vi "Send Initial Position Command.vi"(1 "MCL Command In":refnum<queue>, 2 "Ramp Times":cluster{"Initial":T1, "Iterative":T1}, 3 "error in":errorcluster) -> (5 "MCL Command Out":refnum<queue>, 6 "error out":errorcluster)   [LabVIEW 2009]
uses:
  Mixed Mode Command.ctl
  Mixed Mode Command Action.ctl
  Ramp Time Tuple.ctl
  Target Data.ctl
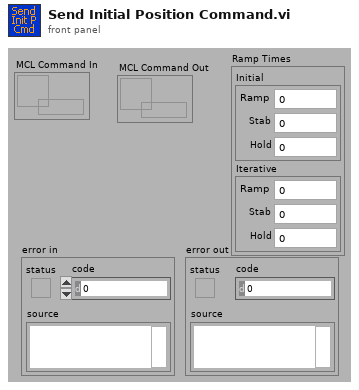
[diagram p1: front panel]
types:
  T1 = typedef "Ramp Time Tuple.ctl" = cluster{"Ramp":dbl, "Stab":dbl, "Hold":dbl}
  T2 = typedef "Mixed Mode Command Action.ctl" = enum16{"Start Command", "Stop", "Exit", "No Op", "Start Acquisition", "Measure Initial Position"}
  T3 = typedef "Mixed Mode Command.ctl" = cluster{"Command":T2, "Ramp Times":cluster{"Initial":T1, "Iterative":T1}, "LBCB1":T4, "LBCB2":T4}
  T4 = typedef "Target Data.ctl" = cluster{"Displacements":dbl[], "Command Type":enum16{"<None>", "Displacement", "Force"}[], "Forces":dbl[]}
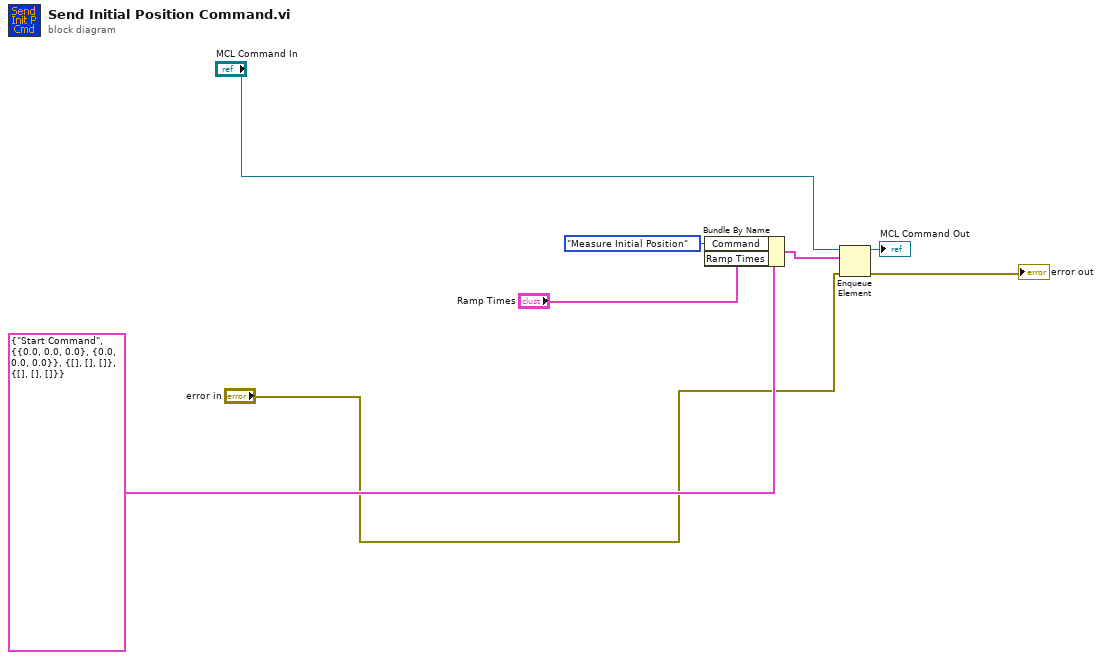
[diagram p0: block diagram]
diagram:
  n1 = Bundle By Name(cluster=T3 {"Command"=enum."Start Command", "Ramp Times"={"Initial"={"Ramp"=0.0, "Stab"=0.0, "Hold"=0.0}, "Iterative"={"Ramp"=0.0, "Stab"=0.0, "Hold"=0.0}}, "LBCB1"={"Displacements"=[], "Command Type"=[], "Forces"=[]}, "LBCB2"={"Displacements"=[], "Command Type"=[], "Forces"=[]}} ("Mixed Mode Command In"), "Command"=Mixed_Mode_Command_Action."Measure Initial Position", "Ramp Times"="Ramp Times") -> (w4:T3)
  n2 = Enqueue Element(queue="MCL Command In", element=w4, error in (no error)="error in") -> (queue out=→"MCL Command Out":refnum<queue>, error out=→"error out":errorcluster)  [unwired: 1 in, 1 out]
